vi "CAN Filter Messages.vi"(7 "Mode":u8, 8 "error in (no error)":errorcluster caption="错误输入（无错误）", 9 "ToID":u32, 10 "FromID":u32, 11 "Channel":u8) -> (0 "error out":errorcluster caption="错误输出", 3 "function return":u32)   [LabVIEW 2021]
doc: "TPCANStatus __stdcall CAN_FilterMessages(\n TPCANHandle Channel, \n DWORD FromID, \n DWORD ToID, \n TPCANMode Mode);"
uses:
  PCANBasic.dll
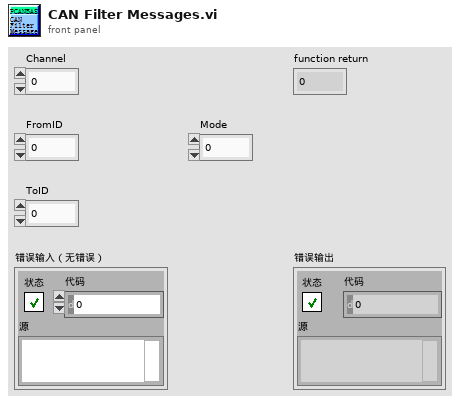
[diagram p1: front panel]
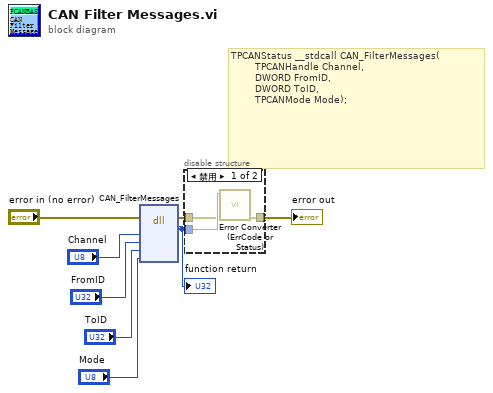
[diagram p0: block diagram]
diagram:
  # "TPCANStatus __stdcall CAN_FilterMessages(\n        TPCANHandle Channel, \n        DWORD FromID, \n        DWORD ToID, \n        TPCANMode Mode);"
  n1 = dll-call lib="D:/ON LINE WORK/LabVIEW/PCAN/PCAN 1.6(2021)/PCANBasic.*" fn="CAN_FilterMessages"(error in="error in (no error)", "Channel"="Channel", "FromID"="FromID", "ToID"="ToID", "Mode"="Mode") -> (error out=w2:errorcluster, "返回类型"=w8:u32)  [unwired: 6 in, 1 out]
  "function return" <- w8
  n2 = disable-structure shown="禁用" {
    disable-tunnel: w8 -> [w11 _]
    disable-tunnel: w2 -> [w10 _]
    disable-tunnel: [w9 _] -> w1
    frame Disabled {
      n3 = call "Error Converter (ErrCode or Status).vi"("error in (no error)"=w10, "error code"=w11) -> ("error out"=w9:errorcluster)  [unwired: 9 in]
    }
    frame Enabled {
    }
  }
  "error out" <- w1
